vi "Poll Position Sensor.vi"(8 "error in (no error)":errorcluster, 11 "Cylinder.lvclass":refnum<class "Cylinder.lvclass">) -> ()   [LabVIEW 2015, in "cRIO-Carbondioxide.lvlib" / "CO2-Actor.lvlib" / "Cylinder.lvclass"]
uses:
  Cylinder.lvclass
  Cylinder.lvclass/Cylinder.ctl
  <vilib>/ptbypt/NI_PtbyPt.lvlib
panel:
  out "error out":errorcluster
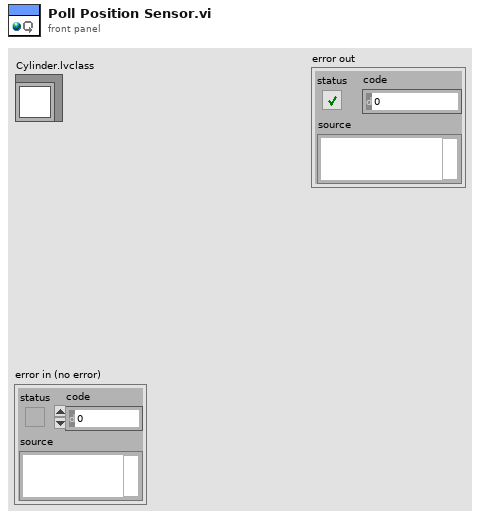
[diagram p1: front panel]
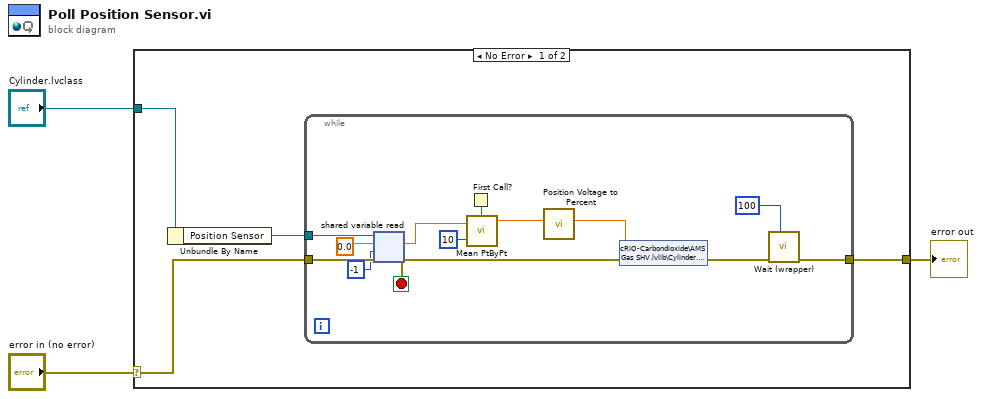
[diagram p0: block diagram]
diagram:
  n1 = case shown="No Error" "error in (no error)" {
    selector: "error in (no error)" -> [w5 w21]
    tunnel: "Cylinder.lvclass" -> [w6 _]
    tunnel: [w4 w21] -> w1
    frame No Error {
      n2 = Unbundle By Name(w6) -> ("Position Sensor"=w7:refnum<k21>)
      n3 = while {
        tunnel: w7 -> [w17]
        tunnel: w5 -> [w20]
        tunnel: [w18] -> w4
        stop <- w12 stop-if-true
        n4 = shared-variable-read(w17, w20, 0.0, -1 ("timeout ms")) -> (w12:errorcluster, w14:dbl)  [unwired: 3 out]
        n5 = First Call?() -> (First Call?: T/F=w15:bool)
        n6 = call <vilib>:"Mean PtByPt.vi"("x"=w14, "sample length"=10, "initialize"=w15) -> ("mean"=w9:dbl)  [unwired: 1 in, 1 out]
        n7 = call "Position Voltage to Percent.vi"("Position Sensor Output (V)"=w9) -> ("Cylinder Position (%)"=w8:dbl)  [unwired: 10 in]
        n8 = shared-variable "cRIO-Carbondioxide\\AMS Gas SHV.lvlib\\Cylinder.lvlib\\Position"(w8, error in=w12) -> (error out=w11:errorcluster)
        n9 = call "Wait (wrapper).vi"("milliseconds to wait (200)"=u32 100, "error in (no error)"=w11) -> ("error out"=w18:errorcluster)  [unwired: 9 in]
      }
    }
    frame Error {
    }
  }
  "error out" <- w1
